vi "open new VI reference.vi"(8 "error in":errorcluster, 11 "UI Reference configuration in":refnum<class "UI Reference configuration.lvclass">) -> (0 "error out":errorcluster, 2 "VI Refnum":refnum<vi>, 3 "UI Reference configuration out":refnum<class "UI Reference configuration.lvclass">)   [LabVIEW 2015, in "UI Reference configuration.lvclass"]
uses:
  UI Reference configuration.lvclass
  UI Reference configuration.lvclass/UI Reference configuration.ctl
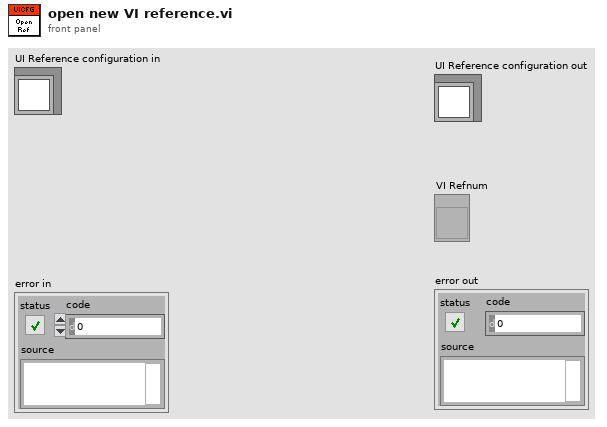
[diagram p1: front panel]
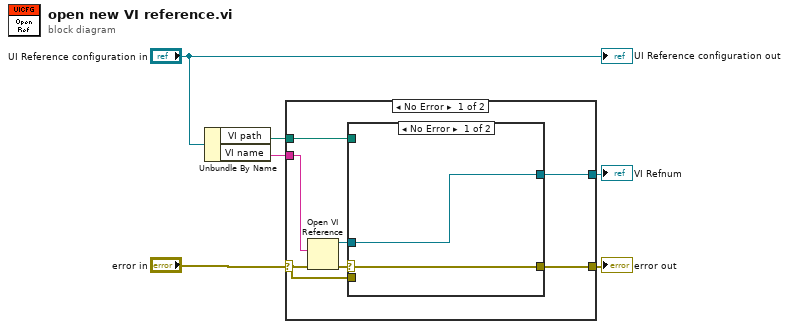
[diagram p0: block diagram]
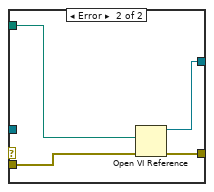
[diagram p2: hidden frame]
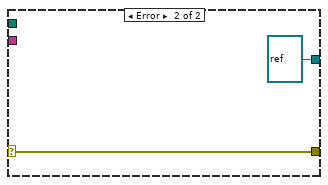
[diagram p3: hidden frame]
diagram:
  n1 = Unbundle By Name("UI Reference configuration in") -> ("VI path"=w5:path, "VI name"=w6:string)
  n2 = case shown="No Error" "error in" {
    selector: "error in" -> [w10 w21]
    tunnel: [w13 refnum<vi> refnum ("VI reference")] -> w3
    tunnel: w6 -> [w12 _]
    tunnel: [w11 w21] -> w2
    tunnel: w5 -> [w7 _]
    frame No Error {
      n3 = Open VI Reference(vi path=w12, error in (no error)=w10) -> (vi reference=w8:refnum<vi>, error out=w9:errorcluster)  [unwired: 4 in]
      n4 = case shown="No Error" w9 {
        selector: w9 -> [w14 _]
        tunnel: [w15 w17] -> w13
        tunnel: w8 -> [w15 _]
        tunnel: [w14 w18] -> w11
        tunnel: w10 -> [_ w19]
        tunnel: w7 -> [_ w16]
        frame No Error {
        }
        frame Error {
          n5 = Open VI Reference(vi path=w16, error in (no error)=w19) -> (vi reference=w17:refnum<vi>, error out=w18:errorcluster)  [unwired: 4 in]
        }
      }
    }
    frame Error {
    }
  }
  "VI Refnum" <- w3
  "error out" <- w2
  "UI Reference configuration out" <- "UI Reference configuration in"
